vi "PnumaticManager.vi"   [LabVIEW 2014]
uses:
  <vilib>/Rock Robotics/WPI/Solenoid/WPI_SolenoidValue.ctl
  Robot Global Data.vi
  <vilib>/Rock Robotics/WPI/Solenoid/WPI_SolenoidSetEnum.vi
types:
  T1 = typedef "WPI_SolenoidValue.ctl" = enum16{"Off", "On", "Forward", "Reverse"}
  T2 = typedef "WPI_SolenoidDevRef.ctl" = cluster{"DevStatus":errorcluster, "Pneumatics Control Module":u8, "Forward Solenoid Channel":T3, "Reverse Solenoid Channel":T3}
  T3 = typedef "WPI_SolenoidChannel.ctl" = enum8{"Solenoid 0", "Solenoid 1", "Solenoid 2", "Solenoid 3", "Solenoid 4", "Solenoid 5", "Solenoid 6", "Solenoid 7", "Invalid"}
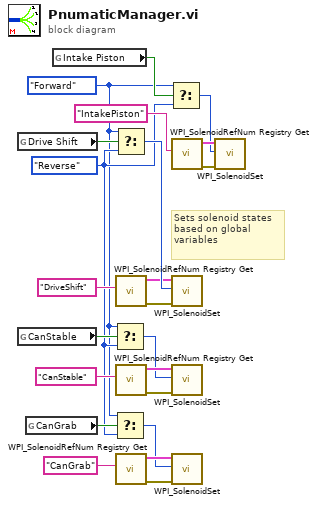
[diagram p0: block diagram]
diagram:
  w4 = WPI_SolenoidValue."Reverse" ("Value")
  w3 = WPI_SolenoidValue."Forward" ("Value")
  # "Sets solenoid states based on global variables"
  n1 = global read "Robot Global Data.vi" "Drive Shift"() -> (w21:bool)
  n2 = global read "Robot Global Data.vi" "CanStable"() -> (w11:bool)
  n3 = global read "Robot Global Data.vi" "CanGrab"() -> (w12:bool)
  n4 = global read "Robot Global Data.vi" "Intake Piston"() -> (w13:bool)
  n5 = Select(t=w3, s=w11, f=w4) -> (s? t:f=w1:T1)
  n6 = Select(t=w3, s=w12, f=w4) -> (s? t:f=w2:T1)
  n7 = Select(t=w3, s=w21, f=w4) -> (s? t:f=w20:T1)
  n8 = call <vilib>:"WPI_SolenoidRefNum Registry Get.vi"("refnum name"="DriveShift") -> ("error out"=w18:errorcluster, "SolenoidDevRef"=w19:T2)  [unwired: 9 in]
  n9 = call <vilib>:"WPI_SolenoidRefNum Registry Get.vi"("refnum name"="CanStable") -> ("error out"=w5:errorcluster, "SolenoidDevRef"=w6:T2)  [unwired: 9 in]
  n10 = call <vilib>:"WPI_SolenoidRefNum Registry Get.vi"("refnum name"="CanGrab") -> ("error out"=w8:errorcluster, "SolenoidDevRef"=w9:T2)  [unwired: 9 in]
  n11 = Select(t=w3, s=w13, f=w4) -> (s? t:f=w14:T1)
  n12 = call <vilib>:"WPI_SolenoidRefNum Registry Get.vi"("refnum name"="IntakePiston") -> ("error out"=w16:errorcluster, "SolenoidDevRef"=w15:T2)  [unwired: 9 in]
  n13 = call-poly <vilib>:"WPI_SolenoidSet.vi"("error in (no error)"=w18, "Value"=w20, "SolenoidDevRef"=w19) -> ()  [unwired: 7 in, 2 out]
  n14 = call-poly <vilib>:"WPI_SolenoidSet.vi"("error in (no error)"=w5, "Value"=w1, "SolenoidDevRef"=w6) -> ()  [unwired: 7 in, 2 out]
  n15 = call-poly <vilib>:"WPI_SolenoidSet.vi"("error in (no error)"=w8, "Value"=w2, "SolenoidDevRef"=w9) -> ()  [unwired: 7 in, 2 out]
  n16 = call-poly <vilib>:"WPI_SolenoidSet.vi"("error in (no error)"=w16, "Value"=w14, "SolenoidDevRef"=w15) -> ()  [unwired: 7 in, 2 out]
